vi "8.1.vi"() -> ()   [LabVIEW 2017]
panel:
  out "format string":string
  out "Numeric 2":i32
  out "Numeric":i32
  out "size(s)":i32
  out "subarray":string[](array[string])
  in  "String":string
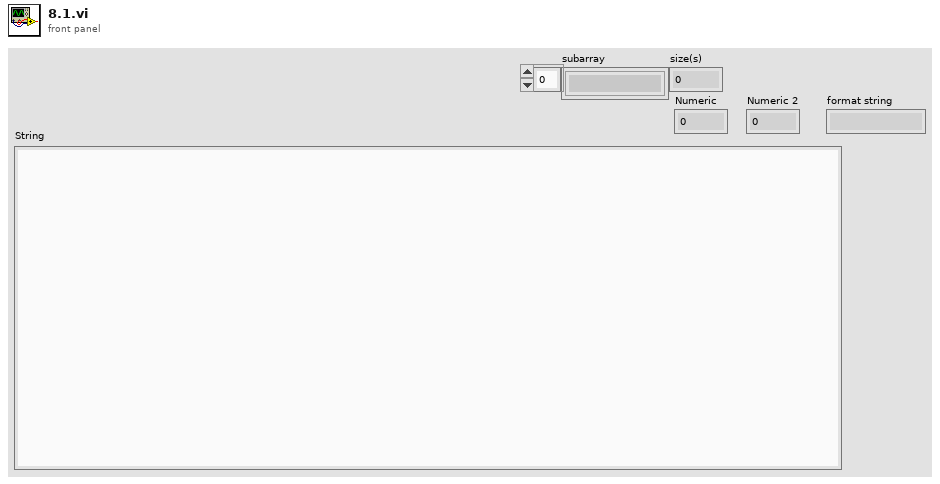
[diagram p1: front panel]
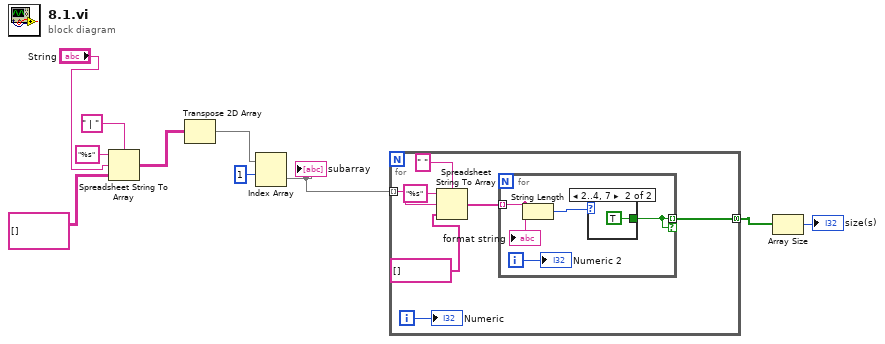
[diagram p0: block diagram]
diagram:
  n1 = Spreadsheet String To Array(delimiter (Tab)=" | ", format string="%s", spreadsheet string="String", array type (2D Dbl)=string[][] []) -> (array=w6:string[][])
  n2 = Transpose 2D Array(2D array=w6) -> (transposed array=w5:string[][])
  n3 = Index Array(array=w5, index (row)=1) -> (element=w3:string[])  [unwired: 1 in]
  "subarray" <- w3
  n4 = for {
    tunnel: w3 -> [w17] mode=indexing
    tunnel: [w12] -> w2 mode=concatenating
    i -> [w11]
    n5 = Spreadsheet String To Array(delimiter (Tab)=" ", format string="%s", spreadsheet string=w17, array type (2D Dbl)=string[] []) -> (array=w13:string[])
    n6 = for {
      tunnel: w13 -> [w21] mode=indexing
      tunnel: [w19] -> w12 mode=indexing if=w19
      i -> [w18]
      n7 = String Length(string=w21) -> (length=w20:i32)
      n8 = case shown="2..4, 7" w20 {
        tunnel: [_ TRUE] -> w19
        frame 0, Default {
        }
        frame 2..4, 7 {
        }
      }
      "Numeric 2" <- w18
      "format string" <- w21
    }
    "Numeric" <- w11
  }
  n9 = Array Size(array=w2) -> (size(s)=→"size(s)":i32)
